vi "LVClass_CameraSet ReadFile CameraParametersSetup.vi"(0 "CameraSet in":refnum<class "CameraSet.lvclass">, 11 "error in (no error)":errorcluster) -> (4 "CameraSet out":refnum<class "CameraSet.lvclass">, 15 "error out":errorcluster)   [LabVIEW 2020, in "CameraSet.lvclass"]
uses:
  CameraSet.lvclass
  CameraSet.lvclass/CameraSet.ctl
  Read From XML File(array).vi
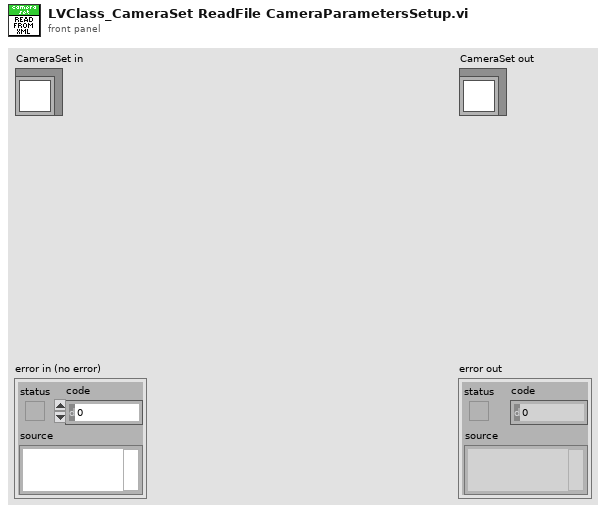
[diagram p1: front panel]
types:
  T1 = typedef "CameraParametersSetup.ctl" = cluster{"Name":string, "Type":T2, "Value":dbl, "BooleanValue":bool, "StringValue":string}
  T2 = typedef "CameraParameters_Type.ctl" = enum16{"Integer", "Real", "String", "Boolean"}
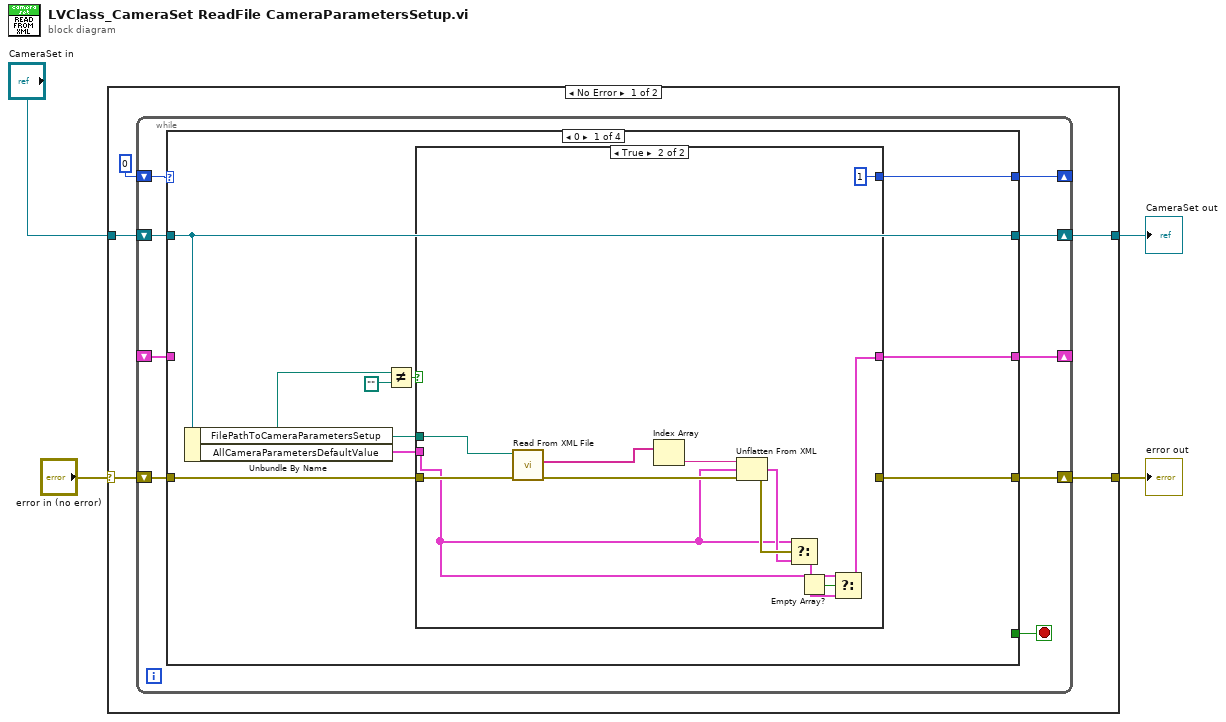
[diagram p0: block diagram]
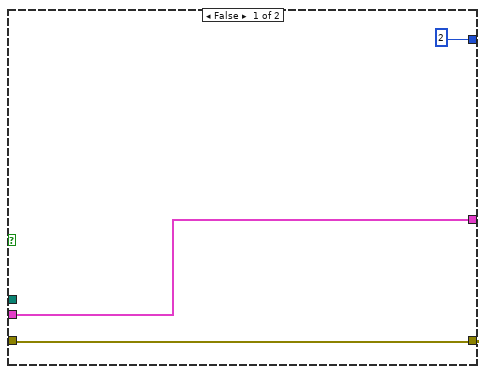
[diagram p2: hidden frame]
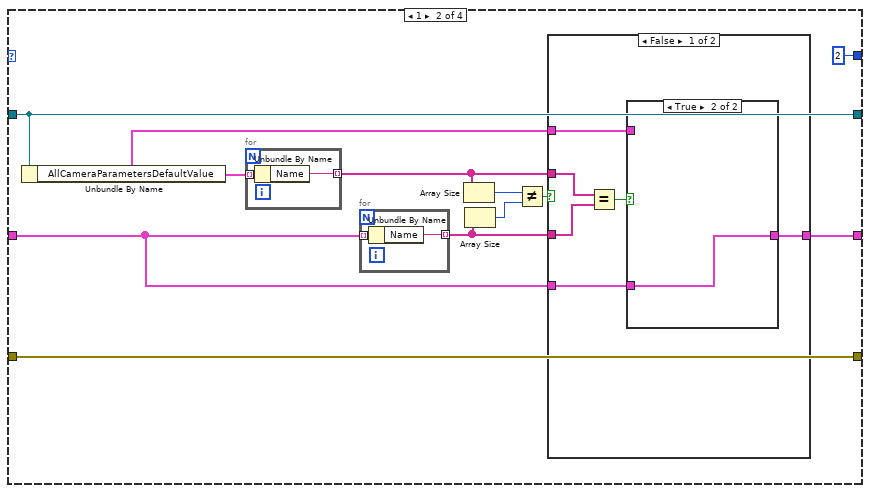
[diagram p3: hidden frame]
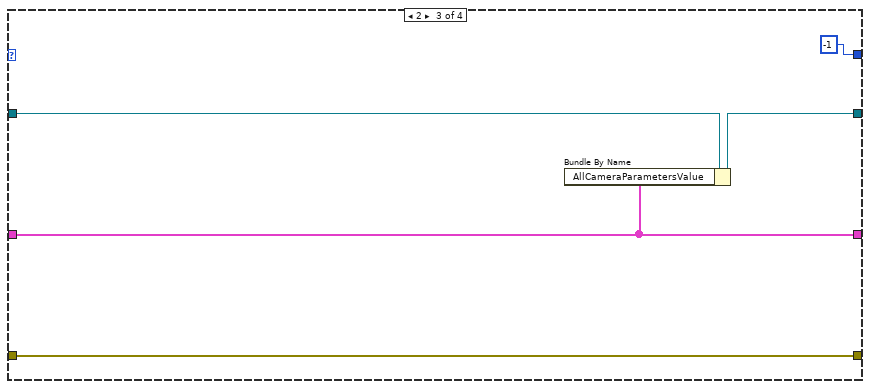
[diagram p6: hidden frame]
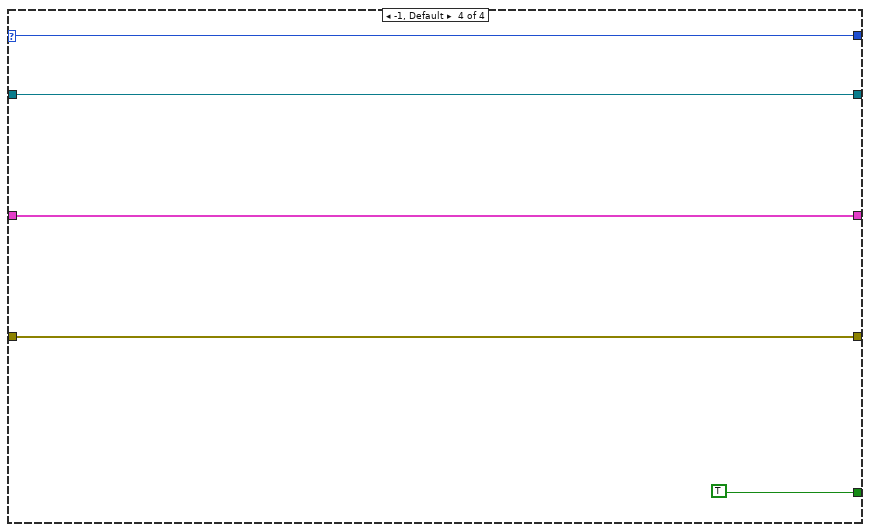
[diagram p7: hidden frame]
diagram:
  n1 = case shown="No Error" "error in (no error)" {
    selector: "error in (no error)" -> [w8 w78]
    tunnel: [w9 w78] -> w3
    tunnel: "CameraSet in" -> [w6 w77]
    tunnel: [w5 w77] -> w1
    frame No Error {
      n2 = while {
        shift-right: [w16] -> _
        shift-left: _ -> [w12]
        shift-right: [w10] -> _
        shift-left: 0 -> [w14]
        shift-right: [w11] -> w5
        shift-left: w6 -> [w15]
        shift-right: [w18] -> w9
        shift-left: w8 -> [w17]
        stop <- w13 stop-if-true
        n3 = case shown="0" w14 {
          selector: w14 -> [_ _ _ w72]
          tunnel: [w27 w43 w67 w75] -> w18
          tunnel: w17 -> [w26 w43 w67 w75]
          tunnel: [w22 w47 w68 w74] -> w16
          tunnel: w15 -> [w20 w52 w71 w73]
          tunnel: [_ _ _ TRUE] -> w13
          tunnel: w12 -> [_ w44 w68 w74]
          tunnel: [w20 w52 w70 w73] -> w11
          tunnel: [w19 2 -1 w72] -> w10
          frame 0 {
            n4 = Unbundle By Name(w20) -> ("FilePathToCameraParametersSetup"=w24:path, "AllCameraParametersDefaultValue"=w21:T1[])
            n5 = Not Equal?(x=w24, y=path "") -> (x != y?=w23:bool)
            n6 = case shown="True" w23 {
              tunnel: w24 -> [_ w39]
              tunnel: [w30 _] -> w27
              tunnel: w26 -> [w30 w38]
              tunnel: [w29 w33] -> w22
              tunnel: w21 -> [w29 w32]
              tunnel: [2 1] -> w19
              frame False {
              }
              frame True {
                n7 = call-poly "Read From XML File.vi"("error in (no error)"=w38, "XML File Path"=w39) -> ("error out"=w42:errorcluster, "XML Elements"=w41:string[])  [unwired: 7 in, 1 out]
                n8 = Index Array(array=w41) -> (element=w40:string)  [unwired: 1 in]
                n9 = Unflatten From XML(xml string=w40, type=w32, error in (no error)=w42) -> (value=w36:T1[], error out=w37:errorcluster)
                n10 = Select(t=w32, s=w37, f=w36) -> (s? t:f=w34:T1[])
                n11 = Empty Array?(array=w34) -> (empty?=w35:bool)
                n12 = Select(t=w32, s=w35, f=w34) -> (s? t:f=w33:T1[])
              }
            }
          }
          frame 1 {
            n13 = Unbundle By Name(w52) -> ("AllCameraParametersDefaultValue"=w48:T1[])
            n14 = for {
              tunnel: w48 -> [w64] mode=indexing
              tunnel: [w63] -> w46 mode=indexing
              n15 = Unbundle By Name(w64) -> ("Name"=w63:string)
            }
            n16 = for {
              tunnel: w44 -> [w66] mode=indexing
              tunnel: [w65] -> w45 mode=indexing
              n17 = Unbundle By Name(w66) -> ("Name"=w65:string)
            }
            n18 = Array Size(array=w46) -> (size(s)=w51:i32)
            n19 = Array Size(array=w45) -> (size(s)=w50:i32)
            n20 = Not Equal?(x=w51, y=w50) -> (x != y?=w49:bool)
            n21 = case shown="False" w49 {
              tunnel: w48 -> [w54 w62]
              tunnel: [w56 w62] -> w47
              tunnel: w46 -> [w59 _]
              tunnel: w45 -> [w58 _]
              tunnel: w44 -> [w55 _]
              frame False {
                n22 = Equal?(x=w59, y=w58) -> (x = y?=w57:bool)
                n23 = case shown="True" w57 {
                  tunnel: [w60 w61] -> w56
                  tunnel: w55 -> [_ w61]
                  tunnel: w54 -> [w60 _]
                  frame False {
                  }
                  frame True {
                  }
                }
              }
              frame True {
              }
            }
          }
          frame 2 {
            n24 = Bundle By Name(cluster=w71, "AllCameraParametersValue"=w68) -> (w70:refnum<class "CameraSet.lvclass">)
          }
          frame -1, Default {
          }
        }
      }
    }
    frame Error {
    }
  }
  "error out" <- w3
  "CameraSet out" <- w1
